vi "XPARTD_BuildDispCmd.vi"(9 "nodeID":string, 10 "device in":string, 11 "xpapath":string) -> (1 "cmd":string, 4 "device out":string)   [LabVIEW 2016]
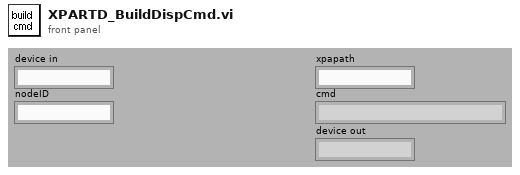
[diagram p1: front panel]
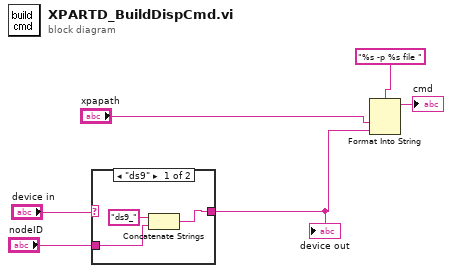
[diagram p0: block diagram]
diagram:
  n1 = case shown="\"ds9\"" "device in" {
    selector: "device in" -> [_ w10]
    tunnel: [w7 w10] -> w3
    tunnel: "nodeID" -> [w8 _]
    frame "ds9" {
      n2 = Concatenate Strings("ds9_" ("string"), w8) -> (w7:string)
    }
    frame Default {
    }
  }
  "device out" <- w3
  n3 = Format Into String(format string="%s -p %s file ", "xpapath", w3) -> (resulting string=→"cmd":string)  [unwired: 2 in, 1 out]
